vi "pp3_trialTypes_selectType.vi"(10 "Trial Type":T2=enum."GO", 11 "Trial Types In":T1[](array[typedef])=[{"Trial Type Number"=1, "Trial Type"=enum."GO", "Trial Weight"=1, "Shock (mA)"=-1.0, "Duration (ms)"=250.0, "Sound Type"=enum."04 FM Sweep", "Stim P1"=2000.0, "Stim P2"=4000.0, "Stim P3"=0.0, "Stim P4"=0.0, "DAQ Amplitude (V)"=0.25}, {"Trial Type Number"=2, "Trial Type"=enum."NOGO", "Trial Weight"=1, "Shock (mA)"=-1.0, "Duration (ms)"=250.0, "Sound Type"=enum."04 FM Sweep", "Stim P1"=4000.0, "Stim P2"=2000.0, "Stim P3"=0.0, "Stim P4"=0.0, "DAQ Amplitude (V)"=0.25}, {"Trial Type Number"=3, "Trial Type"=enum."GO", "Trial Weight"=0, "Shock (mA)"=0.0, "Duration (ms)"=0.0, "Sound Type"=enum."00 NULL", "Stim P1"=0.0, "Stim P2"=0.0, "Stim P3"=0.0, "Stim P4"=0.0, "DAQ Amplitude (V)"=0.25}, {"Trial Type Number"=4, "Trial Type"=enum."TEST", "Trial Weight"=0, "Shock (mA)"=0.0, "Duration (ms)"=0.0, "Sound Type"=enum."00 NULL", "Stim P1"=0.0, "Stim P2"=0.0, "Stim P3"=0.0, "Stim P4"=0.0, "DAQ Amplitude (V)"=0.25}] {"DAQ Amplitude (V)" min=0.0 max=5.0 format="%_4g"; "Shock (mA)" min=-1.0 max=5.0; "Trial Weight" step=1; "Duration (ms)" min=0.0 max=1.0; "Trial Type Number" min=1 max=256 step=1}) -> (0 "Number of Selected Trial Types":i32, 1 "Weight sums":u32, 3 "Trial Types Out":T1[](array[typedef])=[{"Trial Type Number"=1, "Trial Type"=enum."GO", "Trial Weight"=1, "Shock (mA)"=-1.0, "Duration (ms)"=250.0, "Sound Type"=enum."04 FM Sweep", "Stim P1"=2000.0, "Stim P2"=4000.0, "Stim P3"=0.0, "Stim P4"=0.0, "DAQ Amplitude (V)"=0.25}, {"Trial Type Number"=2, "Trial Type"=enum."NOGO", "Trial Weight"=1, "Shock (mA)"=-1.0, "Duration (ms)"=250.0, "Sound Type"=enum."04 FM Sweep", "Stim P1"=4000.0, "Stim P2"=2000.0, "Stim P3"=0.0, "Stim P4"=0.0, "DAQ Amplitude (V)"=0.25}] {"DAQ Amplitude (V)" min=0.0 max=5.0 format="%_4g"; "Shock (mA)" min=-1.0 max=5.0; "Trial Weight" step=1; "Duration (ms)" min=0.0 max=1.0; "Trial Type Number" min=1 max=256 step=1})   [LabVIEW 2013]
uses:
  pp3_CTL_TrialType.ctl
  CTL_pp3g_Trial.ctl
  labolabo2/waveforms/WFTypes.ctl
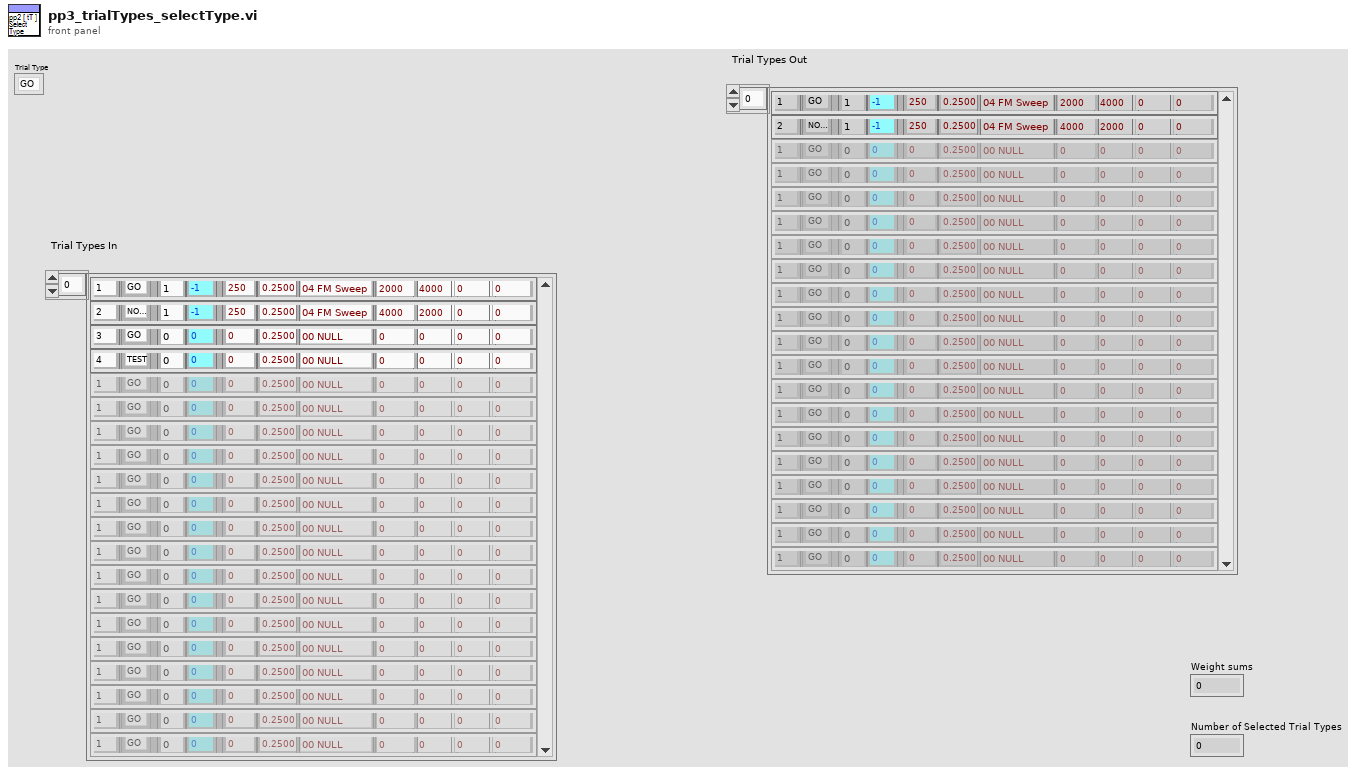
[diagram p1: front panel]
types:
  T1 = typedef "CTL_pp3g_Trial.ctl" = cluster{"Trial Type Number":i16, "Trial Type":T2, "Trial Weight":u32, "Shock (mA)":dbl, "Duration (ms)":dbl, "Sound Type":T3, "Stim P1":dbl, "Stim P2":dbl, "Stim P3":dbl, "Stim P4":dbl, "DAQ Amplitude (V)":dbl}
  T2 = typedef "pp3_CTL_TrialType.ctl" = enum16{"OFF", "GO", "NOGO", "TEST"}
  T3 = typedef "WFTypes.ctl" = enum16{"00 NULL", "01 DC", "02 Noise", "03 Pure Tone", "04 FM Sweep", "05 FM Sweep BURST"}
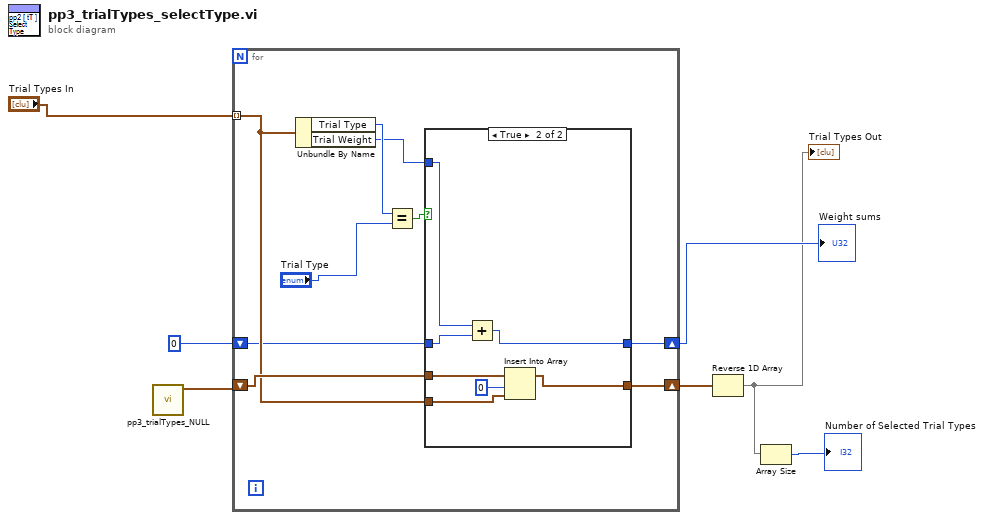
[diagram p0: block diagram]
diagram:
  n1 = call "pp3_trialTypes_NULL.vi"() -> ("Array"=w2:T1[])  [unwired: 11 in]
  n2 = for {
    tunnel: "Trial Types In" -> [w12] mode=indexing
    shift-right: [w13] -> w7
    shift-left: w2 -> [w14]
    shift-right: [w10] -> w4
    shift-left: u32 0 ("Weight sums") -> [w11]
    n3 = Unbundle By Name(w12) -> ("Trial Type"=w16:T2, "Trial Weight"=w9:u32)
    n4 = Equal?(x=w16, y="Trial Type") -> (x = y?=w15:bool)
    n5 = case shown="True" w15 {
      tunnel: w14 -> [w18 w25]
      tunnel: [w18 w24] -> w13
      tunnel: w12 -> [_ w22]
      tunnel: w11 -> [w17 w21]
      tunnel: [w17 w19] -> w10
      tunnel: w9 -> [_ w20]
      frame False {
      }
      frame True {
        n6 = Add(x=w20, y=w21) -> (x+y=w19:u32)
        n7 = Insert Into Array(array=w25, index=0, new element=w22) -> (w24:T1[])
      }
    }
  }
  "Weight sums" <- w4
  n8 = Reverse 1D Array(array=w7) -> (reversed array=w1:T1[])
  "Trial Types Out" <- w1
  n9 = Array Size(array=w1) -> (size(s)=→"Number of Selected Trial Types":i32)
